vi "clear Error.vi"(8 "error in (no error)":errorcluster) -> (0 "error out":errorcluster)   [LabVIEW 2012, in "clearvolume.lvlib"]
doc: "__declspec(dllexport) void __cdecl clearError();"
uses:
  clearvolume.lvlib
  clearvolume.dll
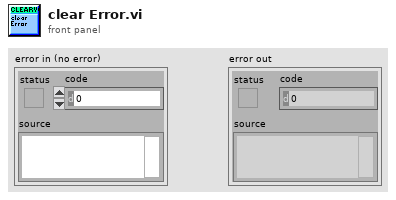
[diagram p1: front panel]
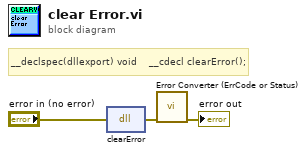
[diagram p0: block diagram]
diagram:
  # "__declspec(dllexport) void \t\t\t__cdecl clearError();"
  n1 = dll-call lib="C:/Users/myerslab/workspace/Libraries/CV/clearvolume/src/labview/clearvolume/clearvolume.*" fn="clearError"(error in="error in (no error)") -> (error out=w2:errorcluster)  [unwired: 3 in, 1 out]
  n2 = call "Error Converter (ErrCode or Status).vi"("error in (no error)"=w2) -> ("error out"=→"error out":errorcluster)  [unwired: 10 in]
